vi "Backup_Client.vi"(1 "Check Updates on Server?":bool, 2 "Get all Server Files":bool, 3 "Months of History to backup":i32) -> (0 "error out":errorcluster)   [LabVIEW 2012]
uses:
  Anemometry/Anemometry Sub Vis/Globals/Preference_global.vi
  Anemometry/Anemometry Sub Vis/Globals/Constants_global.vi
panel:
  out "Array":bool[](array[boolean])
  out "Curnently on":path
  out "Folders to Backup":path[](array[path])
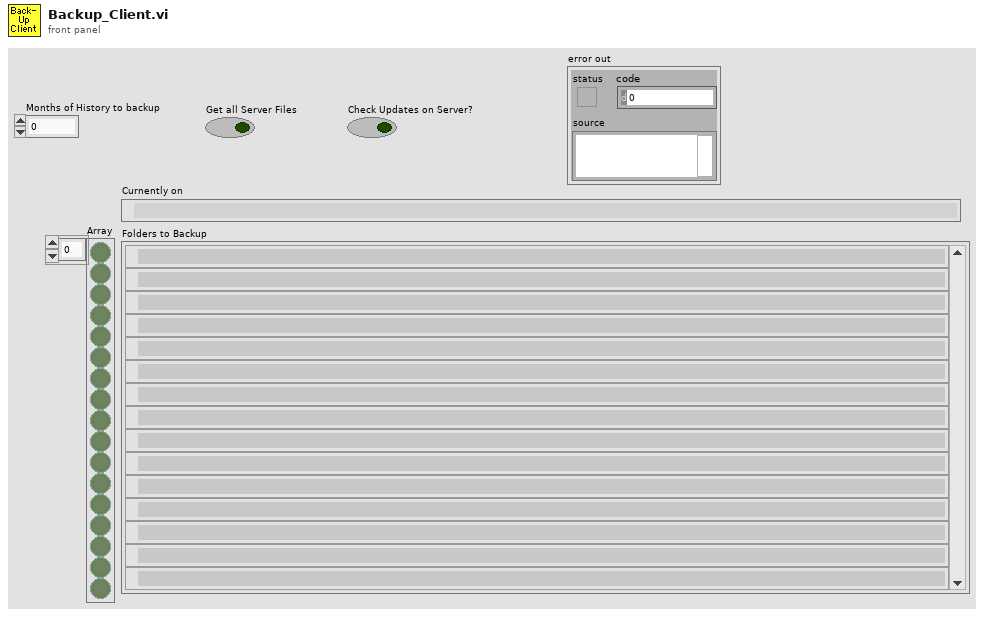
[diagram p1: front panel]
types:
  T1 = typedef "EnFlo_Data_Folder_Setup.ctl" = string
  T2 = typedef "LVDateTimeRec.ctl" = cluster{"fractional second":dbl, "second":i32, "minute":i32, "hour":i32, "day of month":i32, "month":i32, "year":i32, "day of week":i32, "day of year":i32, "DST":i32}
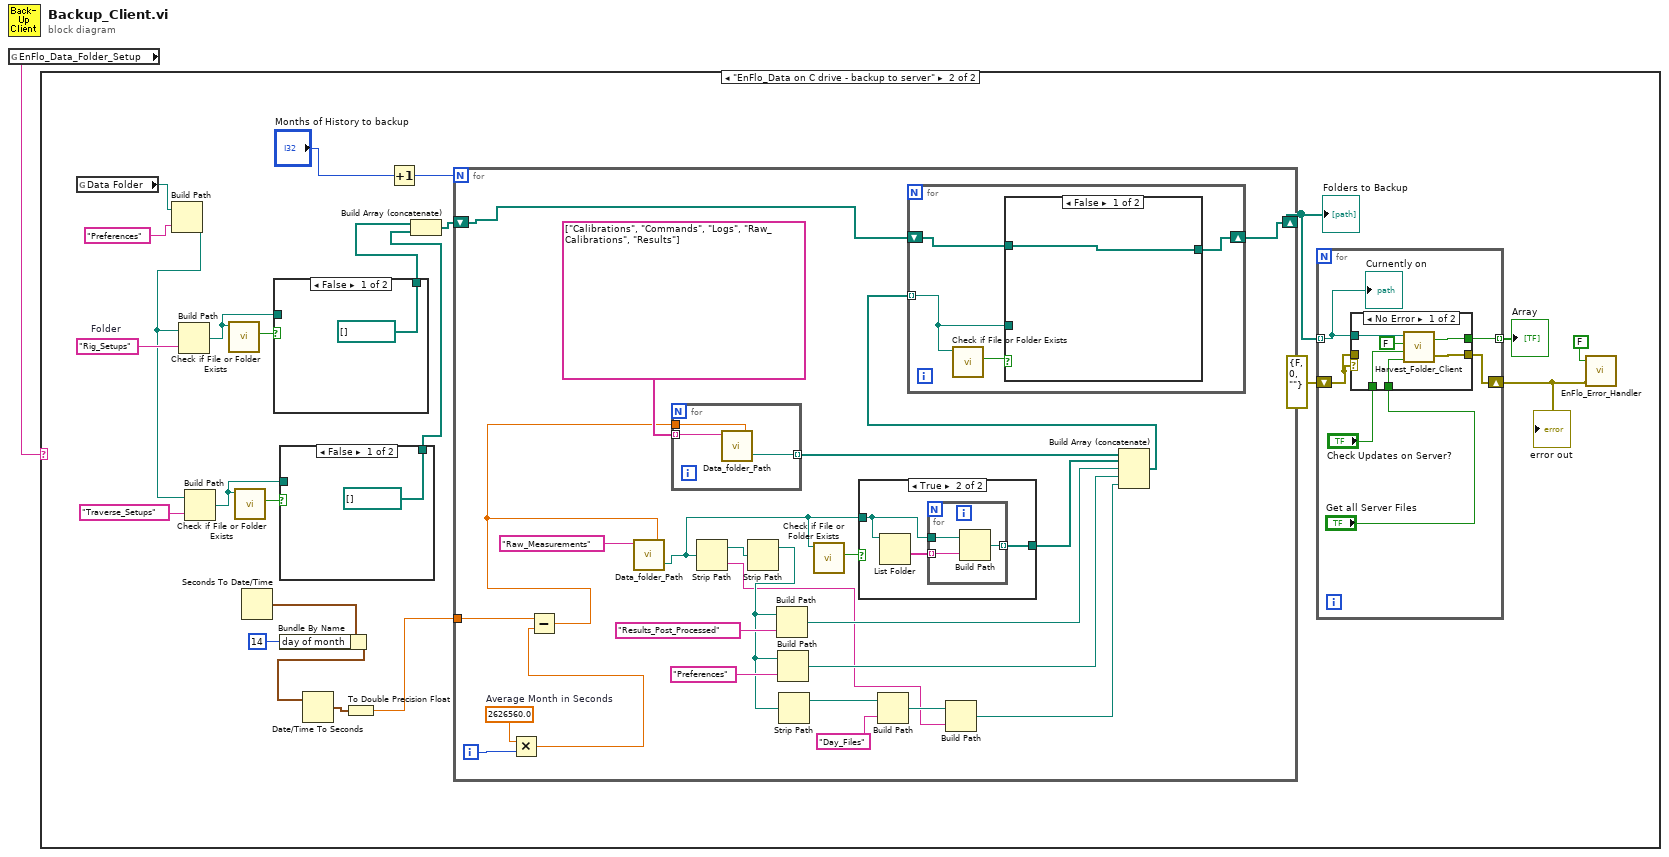
[diagram p0: block diagram]
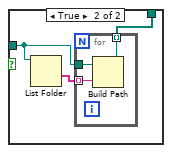
[diagram p3: hidden frame]
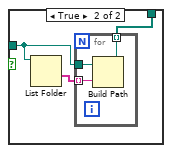
[diagram p4: hidden frame]
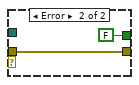
[diagram p5: hidden frame]
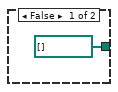
[diagram p6: hidden frame]
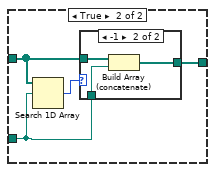
[diagram p7: hidden frame]
diagram:
  n1 = global read "Preference_global.vi" "EnFlo_Data_Folder_Setup"() -> (w1:T1)
  n2 = case shown="\"EnFlo_Data on C drive - backup to server\"" w1 {
    frame "No Match", Default {
    }
    frame "EnFlo_Data on C drive - backup to server" {
      w7 = "Rig_Setups"  # Folder
      n3 = global read "Constants_global.vi" "Data Folder"() -> (w15:path)
      n4 = Build Path(base path=w15, name or relative path="Preferences") -> (appended path=w6:path)
      n5 = Build Path(base path=w6, name or relative path=w7) -> (appended path=w9:path)
      n6 = Build Path(base path=w6, name or relative path="Traverse_Setups") -> (appended path=w10:path)
      n7 = call <vilib>:"Check if File or Folder Exists.vi"("path"=w9) -> ("file or folder exists?"=w8:bool)  [unwired: 8 in, 2 out]
      n8 = call <vilib>:"Check if File or Folder Exists.vi"("path"=w10) -> ("file or folder exists?"=w11:bool)  [unwired: 8 in, 2 out]
      n9 = Seconds To Date/Time() -> (date time rec=w22:T2)  [unwired: 2 in]
      n10 = case shown="False" w8 {
        tunnel: [path[] [] w28] -> w4
        tunnel: w9 -> [_ w27]
        frame False {
        }
        frame True {
          n11 = List Folder(path=w27) -> (folder names=w29:string[])  [unwired: 3 in, 3 out]
          n12 = for {
            tunnel: w29 -> [w32] mode=indexing
            tunnel: w27 -> [w31]
            tunnel: [w30] -> w28 mode=indexing
            n13 = Build Path(base path=w31, name or relative path=w32) -> (appended path=w30:path)
          }
        }
      }
      n14 = case shown="False" w11 {
        tunnel: [path[] [] w35] -> w5
        tunnel: w10 -> [_ w34]
        frame False {
        }
        frame True {
          n15 = List Folder(path=w34) -> (folder names=w36:string[])  [unwired: 3 in, 3 out]
          n16 = for {
            tunnel: w36 -> [w39] mode=indexing
            tunnel: w34 -> [w38]
            tunnel: [w37] -> w35 mode=indexing
            n17 = Build Path(base path=w38, name or relative path=w39) -> (appended path=w37:path)
          }
        }
      }
      n18 = Bundle By Name(cluster=w22, "day of month"=14) -> (w20:T2)
      n19 = Date/Time To Seconds(2:w20) -> (0:w19:timestamp)  [unwired: 1 in]
      n20 = To Double Precision Float(number=w19) -> (double precision float=w23:dbl)
      n21 = Increment(x="Months of History to backup") -> (x+1=w25:i32)
      n22 = Build Array (concatenate)(w4, w5) -> (w13:path[])
      n23 = for {
        N: w25 -> [_]
        tunnel: w23 -> [w68]
        shift-right: [w63] -> w18
        shift-left: w13 -> [w64]
        i -> [w70]
        w71 = 2626560.0  # Average Month in Seconds
        n24 = Multiply(x=w71, y=w70) -> (x*y=w69:dbl)
        n25 = Subtract(x=w68, y=w69) -> (x-y=w67:dbl)
        n26 = call "Data_folder_Path.vi"("seconds"=w67, "Data Type"="Raw_Measurements") -> ("Data Folder"=w62:path)  [unwired: 3 in]
        n27 = for {
          tunnel: string[] ["Calibrations", "Commands", "Logs", "Raw_Calibrations", "Results"] ("appended array") -> [w101] mode=indexing
          tunnel: [w100] -> w77 mode=indexing
          tunnel: w67 -> [w99]
          n28 = call "Data_folder_Path.vi"("seconds"=w99, "Data Type"=w101) -> ("Data Folder"=w100:path)  [unwired: 3 in]
        }
        n29 = Strip Path(path=w62) -> (stripped path=w66:path, name=w55:string)
        n30 = Strip Path(path=w66) -> (stripped path=w59:path)  [unwired: 1 out]
        n31 = Build Path(base path=w59, name or relative path="Results_Post_Processed") -> (appended path=w73:path)
        n32 = Build Path(base path=w59, name or relative path="Preferences") -> (appended path=w60:path)
        n33 = Strip Path(path=w59) -> (stripped path=w58:path)  [unwired: 1 out]
        n34 = call <vilib>:"Check if File or Folder Exists.vi"("path"=w62) -> ("file or folder exists?"=w61:bool)  [unwired: 8 in, 2 out]
        n35 = case shown="True" w61 {
          tunnel: [path[] [] w81] -> w72
          tunnel: w62 -> [_ w80]
          frame False {
          }
          frame True {
            n36 = List Folder(path=w80) -> (folder names=w82:string[])  [unwired: 3 in, 3 out]
            n37 = for {
              tunnel: w82 -> [w85] mode=indexing
              tunnel: w80 -> [w84]
              tunnel: [w83] -> w81 mode=indexing
              n38 = Build Path(base path=w84, name or relative path=w85) -> (appended path=w83:path)
            }
          }
        }
        n39 = Build Path(base path=w58, name or relative path="Day_Files") -> (appended path=w56:path)
        n40 = Build Path(base path=w56, name or relative path=w55) -> (appended path=w54:path)
        n41 = Build Array (concatenate)(w77, w72, w73, w60, w54) -> (w65:path[])
        n42 = for {
          shift-right: [w88] -> w63
          shift-left: w64 -> [w89]
          tunnel: w65 -> [w87] mode=indexing
          n43 = call <vilib>:"Check if File or Folder Exists.vi"("path"=w87) -> ("file or folder exists?"=w86:bool)  [unwired: 8 in, 2 out]
          n44 = case shown="False" w86 {
            tunnel: w89 -> [w90 w93]
            tunnel: w87 -> [_ w92]
            tunnel: [w90 w94] -> w88
            frame False {
            }
            frame True {
              n45 = Search 1D Array(1D array=w93, element=w92) -> (index of element=w91:i32)  [unwired: 1 in]
              n46 = case shown="-1" w91 {
                tunnel: w93 -> [w95 w98]
                tunnel: [w95 w97] -> w94
                tunnel: w92 -> [_ w96]
                frame 0, Default {
                }
                frame -1 {
                  n47 = Build Array (concatenate)(w98, w96) -> (w97:path[])
                }
              }
            }
          }
        }
      }
      "Folders to Backup" <- w18
      n48 = for {
        tunnel: w18 -> [w45] mode=indexing
        tunnel: [w44] -> w17 mode=indexing
        shift-right: [w41] -> w3
        shift-left: errorcluster {"status"=FALSE, "code"=0, "source"=""} ("error out") -> [w40]
        n49 = case shown="No Error" w40 {
          tunnel: w45 -> [w51 _]
          tunnel: [w50 FALSE ("Folder contents changed?")] -> w44
          tunnel: "Check Updates on Server?" -> [w49 _]
          tunnel: "Get all Server Files" -> [w48 _]
          tunnel: [w47 w53] -> w41
          tunnel: w40 -> [_ w53]
          frame No Error {
            n50 = call "Harvest_Folder_Client.vi"("Get all Server Files"=w48, "Check Updates on Server?"=w49, "Archive Files?"=FALSE, "Folder to Harvest"=w51) -> ("error out"=w47:errorcluster, "Folder contents changed?"=w50:bool)  [unwired: 2 out]
          }
          frame Error {
          }
        }
        "Curnently on" <- w45
      }
      "Array" <- w17
      "error out" <- w3
      n51 = call "EnFlo_Error_Handler.vi"("error in (no error)"=w3, "Dialog Box (T)"=FALSE) -> ()  [unwired: 1 in, 3 out]
    }
  }
